vi "ProbabilityRandom.vi"() -> (1 "element":i32)   [LabVIEW 2013]
panel:
  out "nearest integer value":dbl
  out "size(s)":i32
  out "output array":dbl[](array[numeric])
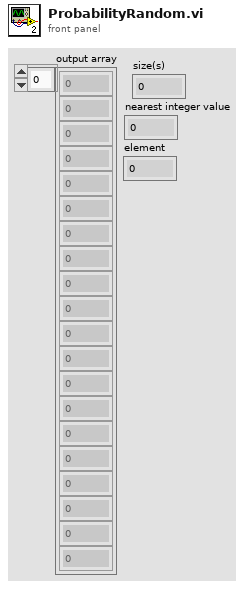
[diagram p1: front panel]
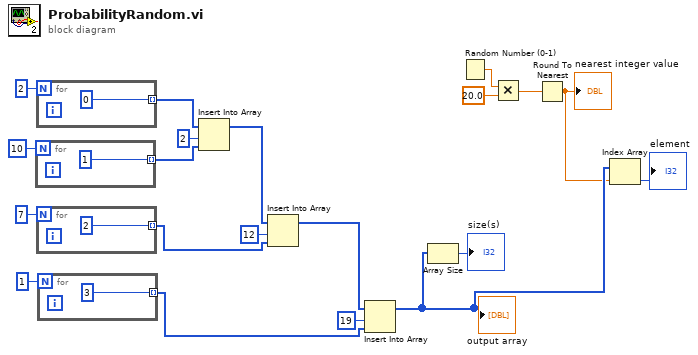
[diagram p0: block diagram]
diagram:
  n1 = for {
    N: 10 -> [_]
    tunnel: [1] -> w16 mode=indexing
  }
  n2 = for {
    N: 2 -> [_]
    tunnel: [0] -> w7 mode=indexing
  }
  n3 = for {
    N: 7 -> [_]
    tunnel: [2] -> w12 mode=indexing
  }
  n4 = for {
    N: 1 -> [_]
    tunnel: [3] -> w10 mode=indexing
  }
  n5 = Insert Into Array(array=w7, index=2, new element=w16) -> (w13:i32[])
  n6 = Insert Into Array(array=w13, index=12, new element=w12) -> (w11:i32[])
  n7 = Insert Into Array(array=w11, index=19, new element=w10) -> (w3:i32[])
  "output array" <- w3
  n8 = Array Size(array=w3) -> (size(s)=→"size(s)":i32)
  n9 = Random Number (0-1)() -> (number: 0 to 1=w4:dbl)
  n10 = Multiply(x=w4, y=20.0) -> (x*y=w5:dbl)
  n11 = Round To Nearest(number=w5) -> (nearest integer value=w2:dbl)
  "nearest integer value" <- w2
  n12 = Index Array(array=w3, index=w2) -> (element=→"element":i32)
